vi "Get Reference for Demodulation.vi"(0 "AI Block Size":i32=5000, 1 "Signal":dbl[][](array[numeric])=array6x5000[30000 elements], 5 "AI Rate":dbl=10000.0 format="%.2f", 7 "OSC Configuration":T3(array[cluster])=[[{"Signal Type"=enum."Sine Wave", "DC"=0.0, "Amplitude"=0.01, "frequency"=2.0, "Phase"=0.0}, {"Signal Type"=enum."Sine Wave", "DC"=0.0, "Amplitude"=0.01, "frequency"=2.0, "Phase"=0.0}], [{"Signal Type"=enum."Sine Wave", "DC"=0.0, "Amplitude"=0.01, "frequency"=2.0, "Phase"=0.0}, {"Signal Type"=enum."Sine Wave", "DC"=0.0, "Amplitude"=0.01, "frequency"=2.0, "Phase"=0.0}]] {"frequency" step=0.001 format="%.3p"; "Amplitude" format="%0.2p"; "DC" min=-0.99 max=0.99 format="%.2p"}, 9 "Phase&Tc":T1(array[cluster])=[{"Phase"=0.0, "Time constant"=0.1, "Set Tc"=FALSE, "Autophase"=FALSE, "Order"=2.0}, {"Phase"=0.0, "Time constant"=0.1, "Set Tc"=FALSE, "Autophase"=FALSE, "Order"=2.0}, {"Phase"=0.0, "Time constant"=0.1, "Set Tc"=FALSE, "Autophase"=FALSE, "Order"=2.0}, {"Phase"=0.0, "Time constant"=0.1, "Set Tc"=FALSE, "Autophase"=FALSE, "Order"=2.0}, {"Phase"=0.0, "Time constant"=0.1, "Set Tc"=FALSE, "Autophase"=FALSE, "Order"=2.0}, {"Phase"=0.0, "Time constant"=0.1, "Set Tc"=FALSE, "Autophase"=FALSE, "Order"=2.0}, {"Phase"=0.0, "Time constant"=0.1, "Set Tc"=FALSE, "Autophase"=FALSE, "Order"=2.0}, {"Phase"=0.0, "Time constant"=0.1, "Set Tc"=FALSE, "Autophase"=FALSE, "Order"=2.0}, {"Phase"=0.0, "Time constant"=0.1, "Set Tc"=FALSE, "Autophase"=FALSE, "Order"=2.0}, {"Phase"=0.0, "Time constant"=0.1, "Set Tc"=FALSE, "Autophase"=FALSE, "Order"=2.0}, {"Phase"=0.0, "Time constant"=0.1, "Set Tc"=FALSE, "Autophase"=FALSE, "Order"=2.0}, {"Phase"=0.0, "Time constant"=0.1, "Set Tc"=FALSE, "Autophase"=FALSE, "Order"=2.0}, {"Phase"=0.0, "Time constant"=0.1, "Set Tc"=FALSE, "Autophase"=FALSE, "Order"=2.0}] {"Phase" min=0.0 max=360.0 scale=0.0..360.0}, 11 "phase log":dbl[](array[numeric])=[0.99999999999938, 0.99999999999938], 12 "Results":dbl[][](array[numeric])=[[-0.007466313257110502, 0.006647442288790556, 0.009996715592438601, 138.3205414893834], [4.666416897873004e-05, 2.73365354254356e-05, 5.408170518337571e-05, 30.36238005772962], [4.0726992829495153e-05, 2.9330066584266565e-05, 5.01890501082782e-05, 35.760031216297186], [4.1405700938166546e-05, 2.8678109848811026e-05, 5.0367311370385436e-05, 34.706961203452664], [4.151375450731611e-05, 2.7252363446332437e-05, 4.965967304266818e-05, 33.28353283261694], [4.150189344545443e-05, 2.848421770375026e-05, 5.033644621695589e-05, 34.463187057405904]]) -> (6 "Ref In":T2(array[cluster]), 8 "Phase Log Out":dbl[](array[numeric]), 10 "Phase&Tc Out":T1(array[cluster]))   [LabVIEW 2013]
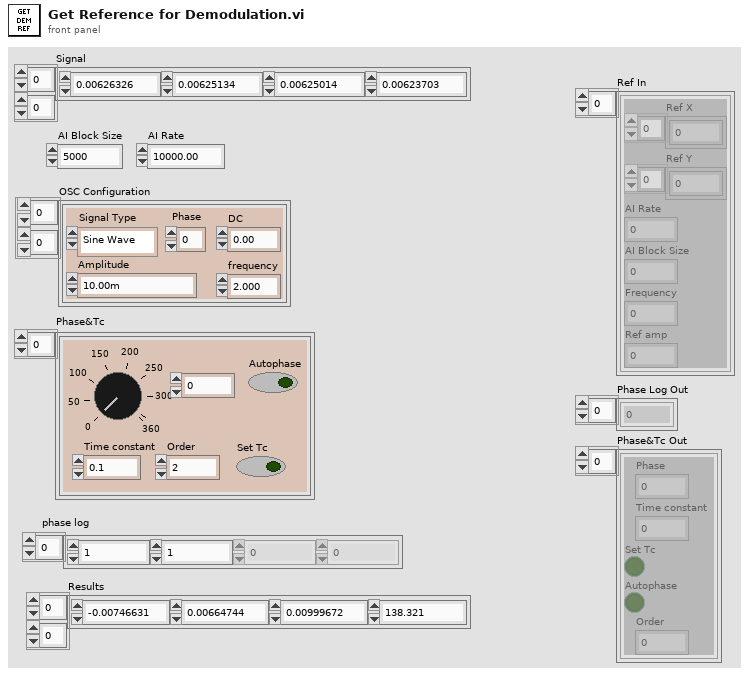
[diagram p1: front panel]
types:
  T1 = cluster{"Phase":dbl, "Time constant":dbl, "Set Tc":bool, "Autophase":bool, "Order":dbl}[]
  T2 = cluster{"Ref X":dbl[], "Ref Y":dbl[], "AI Rate":dbl, "AI Block Size":dbl, "Frequency":dbl, "Ref amp":dbl}[]
  T3 = cluster{"Signal Type":enum16{"Sine Wave", "Triangle Wave", "Square Wave", "Sawtooth Wave"}, "DC":dbl, "Amplitude":dbl, "frequency":dbl, "Phase":dbl}[][]
  T4 = cluster{"Signal Type":enum16{"Sine Wave", "Triangle Wave", "Square Wave", "Sawtooth Wave"}, "DC":dbl, "Amplitude":dbl, "frequency":dbl, "Phase":dbl}
  T5 = cluster{"Ref X":dbl[], "Ref Y":dbl[], "AI Rate":dbl, "AI Block Size":dbl, "Frequency":dbl, "Ref amp":dbl}
  T6 = cluster{"Phase":dbl, "Time constant":dbl, "Set Tc":bool, "Autophase":bool, "Order":dbl}
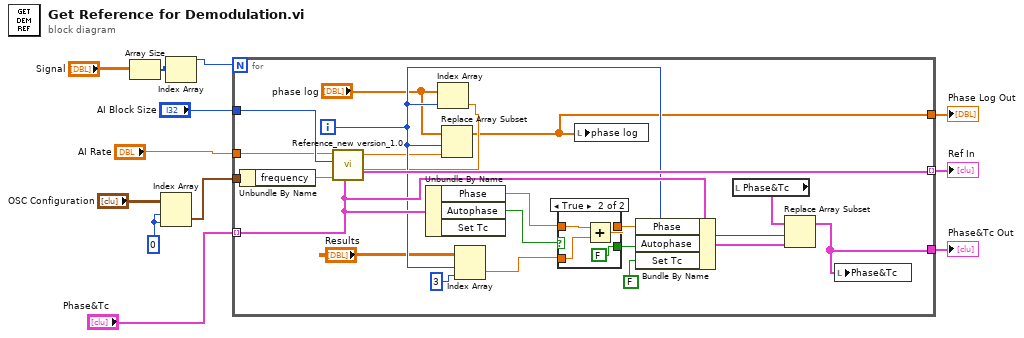
[diagram p0: block diagram]
diagram:
  w7 = 0 ("disabled index (col)")
  n1 = Array Size(array="Signal") -> (size(s)=w11:i32[])
  n2 = Index Array(array="OSC Configuration", index (row)=w7, index (col)=w7) -> (element=w8:T4)
  n3 = Index Array(array=w11) -> (element=w10:i32)  [unwired: 1 in]
  n4 = for {
    N: w10 -> [_]
    tunnel: w8 -> [w34]
    tunnel: "Phase&Tc" -> [w28] mode=indexing
    tunnel: [w32] -> w12 mode=indexing
    tunnel: "AI Block Size" -> [w19]
    tunnel: "AI Rate" -> [w18]
    tunnel: [w15] -> w2
    tunnel: [w13] -> w1
    i -> [w21]
    n5 = Unbundle By Name(w34) -> ("frequency"=w33:dbl)
    n6 = Unbundle By Name(w28) -> ("Phase"=w30:dbl, "Autophase"=w26:bool)  [unwired: 1 out]
    n7 = Index Array(array="phase log", index=w21) -> (element=w17:dbl)
    n8 = call "Reference_new version_1.0.vi"("Phase log in"=w17, "AI Block Size"=w19, "Phase&time"=w28, "Frequency"=w33, "AI Rate"=w18) -> ("Ref out"=w32:T5, "Phase log"=w20:dbl)  [unwired: 3 in]
    n9 = Replace Array Subset(array="phase log", new element=w20, index=w21) -> (w15:dbl[])
    n10 = Index Array(array="Results", index (row)=w21, index (col)=3 ("disabled index (col)")) -> (element=w29:dbl)
    n11 = case shown="True" w26 {
      selector: w26 -> [w35 _]
      tunnel: w30 -> [w36 w40]
      tunnel: w29 -> [_ w37]
      tunnel: [w36 w39] -> w27
      tunnel: [w35 FALSE] -> w25
      frame False {
      }
      frame True {
        n12 = Add(x=w40, y=w37) -> (x+y=w39:dbl)
      }
    }
    n13 = local write "phase log"(w15) -> ()
    n14 = Bundle By Name(cluster=w28, "Phase"=w27, "Autophase"=w25, "Set Tc"=FALSE) -> (w23:T6)
    n15 = local read "Phase&Tc"() -> (w24:T1)
    n16 = Replace Array Subset(array=w24, new element=w23, index=w21) -> (w13:T1)
    n17 = local write "Phase&Tc"(w13) -> ()
  }
  "Ref In" <- w12
  "Phase Log Out" <- w2
  "Phase&Tc Out" <- w1
